vi "Update_UI.vi"(8 "error in (no error)":errorcluster, 10 "data received":string, 11 "Test_Caller in":refnum<class "Test_Caller.lvclass">) -> (0 "error out":errorcluster, 3 "Test_Caller out":refnum<class "Test_Caller.lvclass">)   [LabVIEW 2025, in "Test_Caller.lvlib" / "Test_Caller.lvclass"]
uses:
  Test_Caller.lvclass
  Test_Caller.lvclass/Test_Caller.ctl
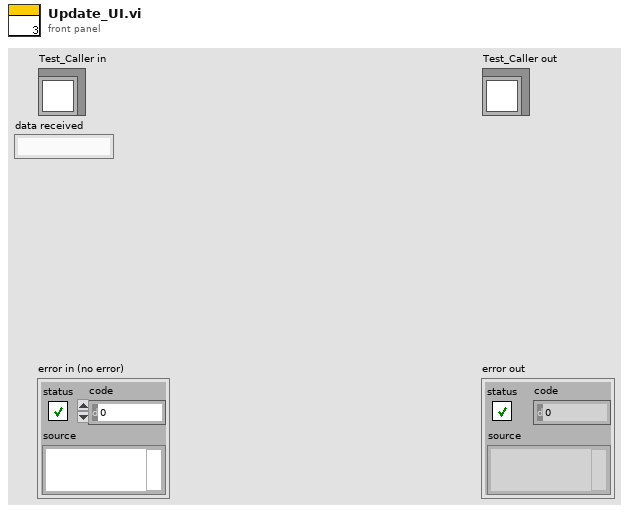
[diagram p1: front panel]
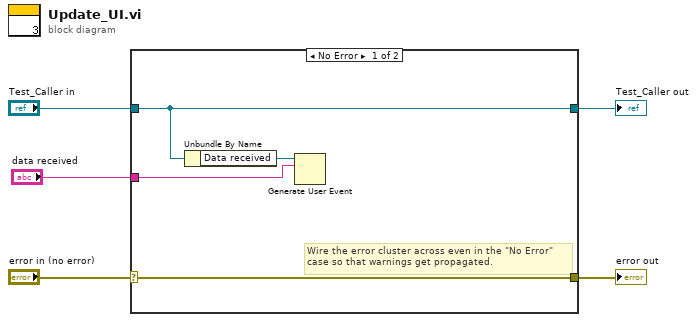
[diagram p0: block diagram]
diagram:
  n1 = case shown="No Error" "error in (no error)" {
    selector: "error in (no error)" -> [w9 w11]
    tunnel: [w9 w11] -> w4
    tunnel: [w8 w10] -> w2
    tunnel: "Test_Caller in" -> [w8 w10]
    tunnel: "data received" -> [w6 _]
    frame No Error {
      # "Wire the error cluster across even in the \"No Error\"\ncase so that warnings get propagated."
      n2 = Unbundle By Name(w8) -> ("Data received"=w7:refnum<user-event>)
      n3 = Generate User Event(user event=w7, event data cluster=w6) -> ()  [unwired: 2 in, 2 out]
    }
    frame Error {
    }
  }
  "error out" <- w4
  "Test_Caller out" <- w2
